vi "Usermgt.vi"(8 "error In":errorcluster) -> (0 "error out":errorcluster)   [LabVIEW 2015]
uses:
  Um- Save.ctl
  Um-Delete.ctl
  Um-Exit.ctl
  <vilib>/addons/database/Connection.llb/DB Tools Open Connec (String).vi
  <vilib>/addons/database/_DB Variant To Data/Database Variant To Data.xnode
  <vilib>/addons/database/NI_Database_API.lvlib
panel:
  out "data":variant[][](array[variant])
  in  "Operator Code":string
  out "error out 3":errorcluster
  out "User Name 2":string
  out "error out 2":errorcluster
  in  "Exit":T1
  in  "Deleat":T2
  in  "Save":T3
  in  "User Type":string
  in  "User Type":u16(ring) items=["Operator", "Supervisor", "admin"]
  in  "Re-Password":string
  in  "Password":string
  in  "User Name":string
  in  "User Table":i32(listbox)
  # "User Create"
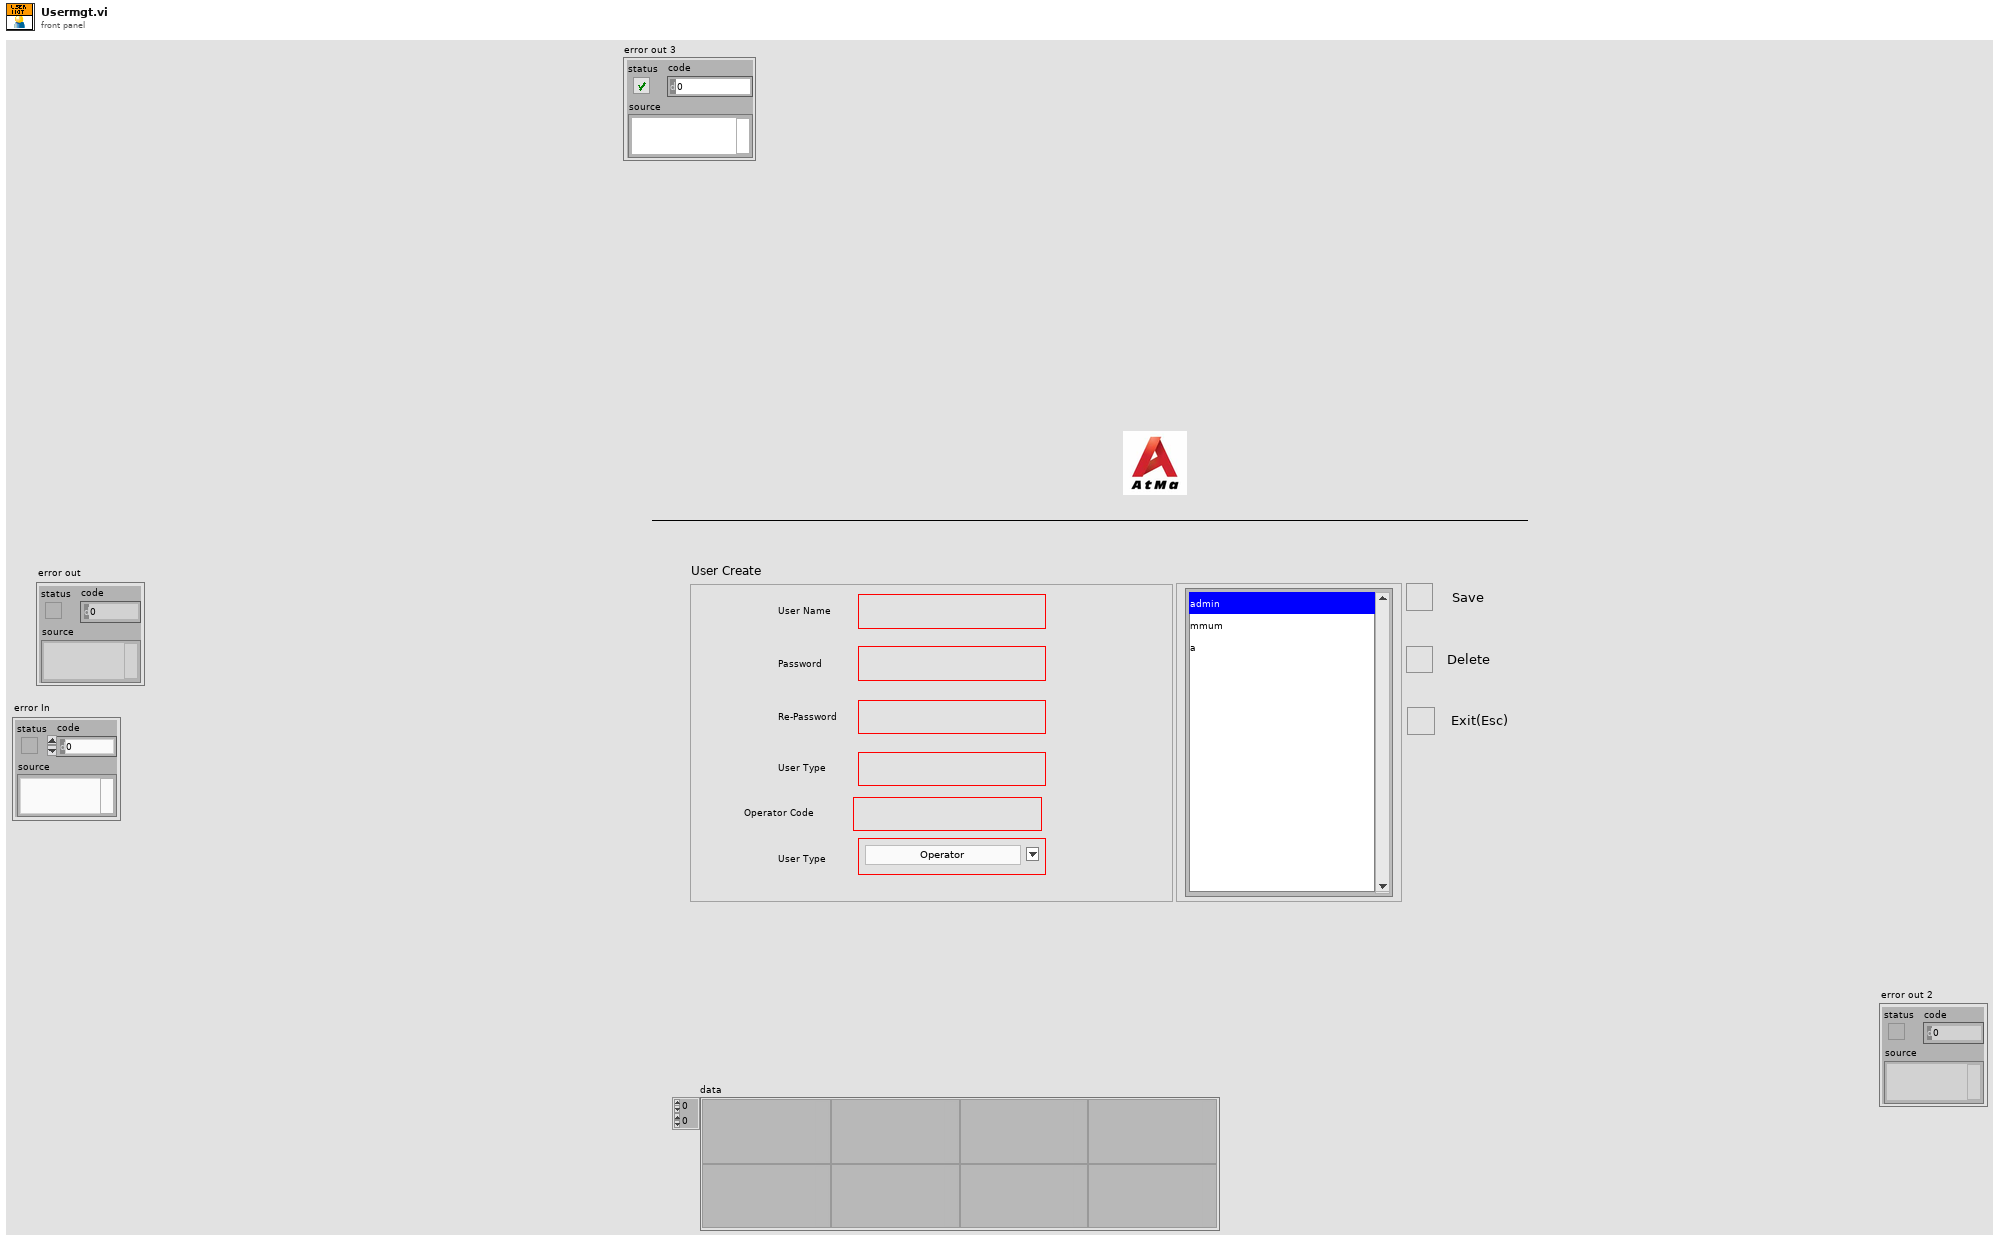
[diagram p1: front panel]
types:
  T1 = typedef "Um-Exit.ctl" = bool
  T2 = typedef "Um-Delete.ctl" = bool
  T3 = typedef "Um- Save.ctl" = bool
  T4 = cluster{"User Name":string, "Password":string, "User Type":string}
  T5 = typedef "NI_Database_API.lvlib/Conn ObjectReference.ctl" = refnum<k1>
  T6 = cluster{"User Name":string, "Password":string, "User Type":string, "Access right":string}
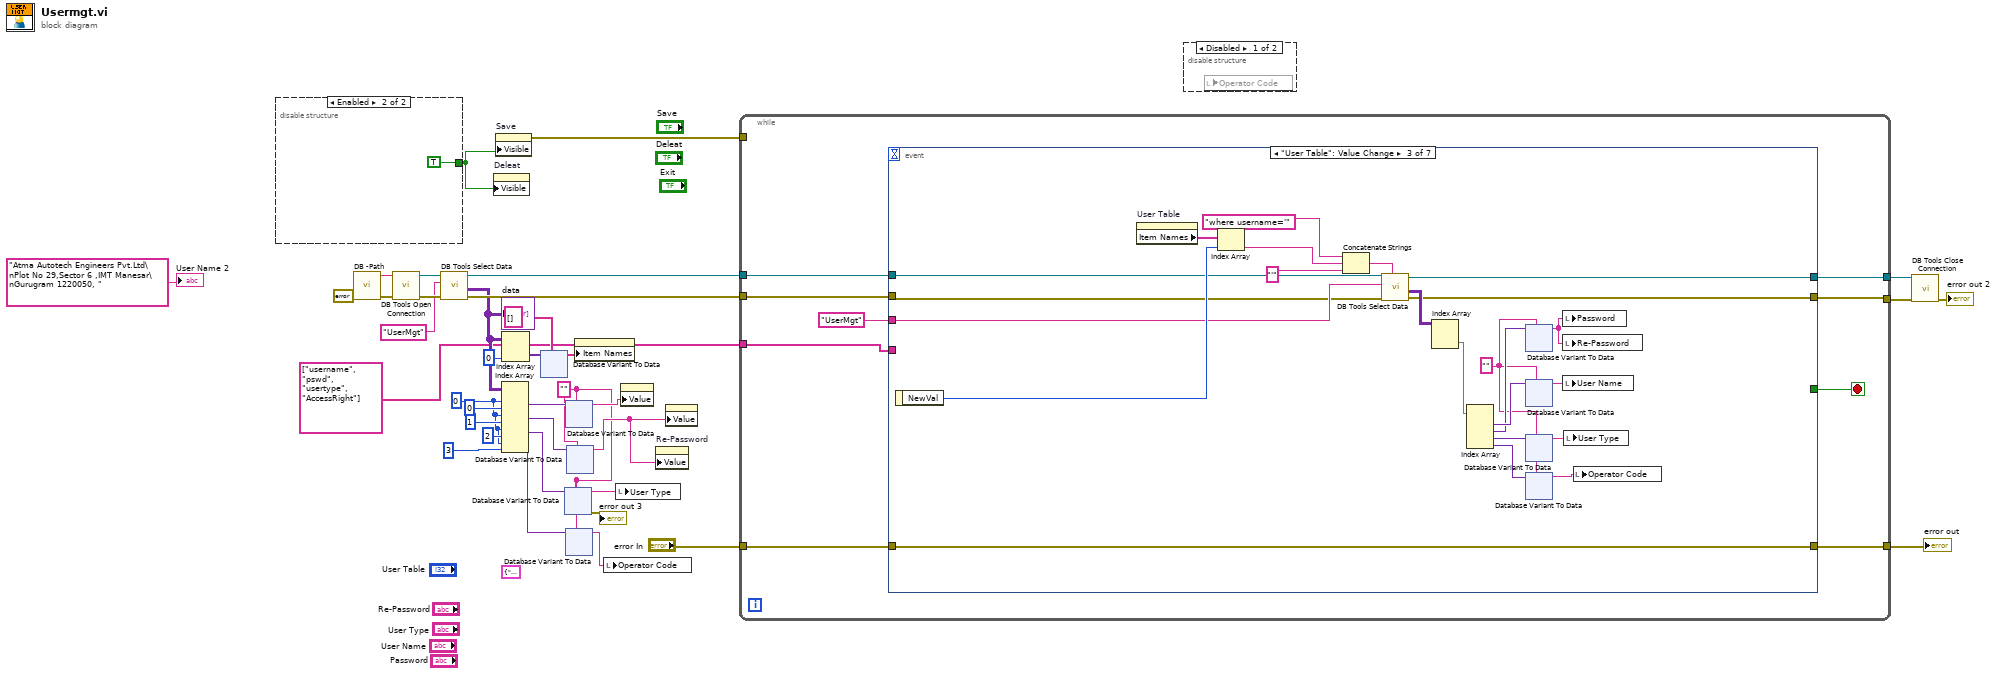
[diagram p0: block diagram]
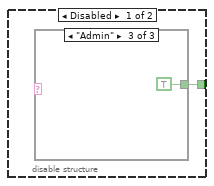
[diagram p3: hidden frame]
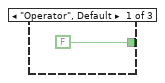
[diagram p4: hidden frame]
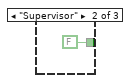
[diagram p5: hidden frame]
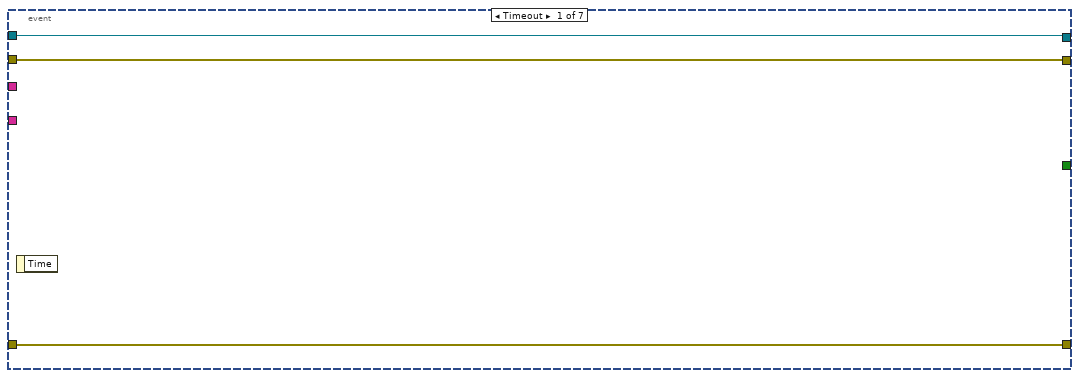
[diagram p6: hidden frame]
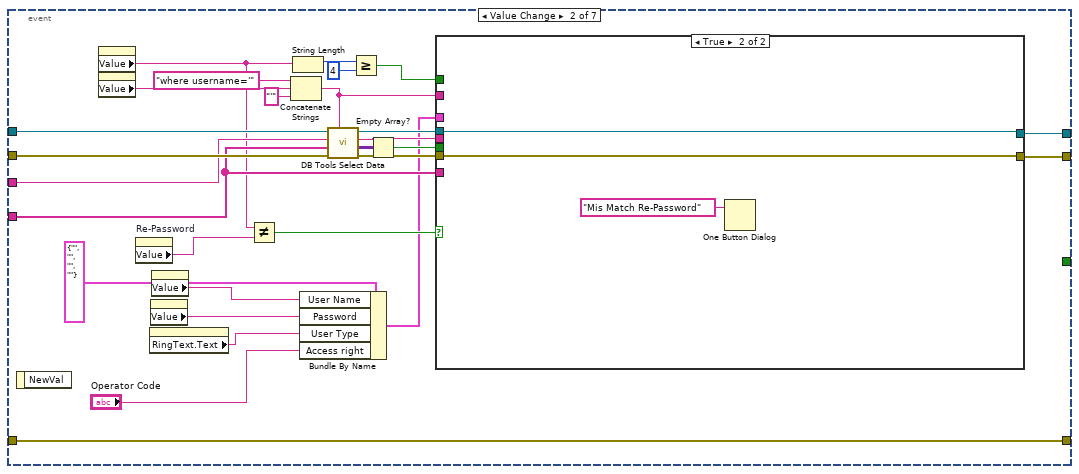
[diagram p7: hidden frame]
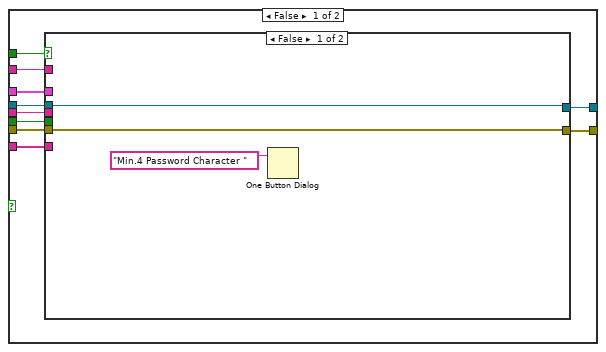
[diagram p8: hidden frame]
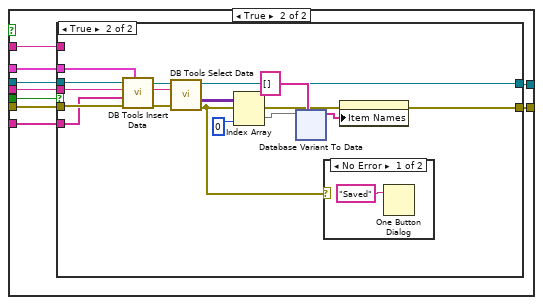
[diagram p9: hidden frame]
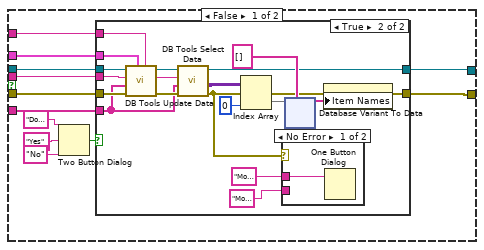
[diagram p10: hidden frame]
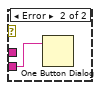
[diagram p12: hidden frame]
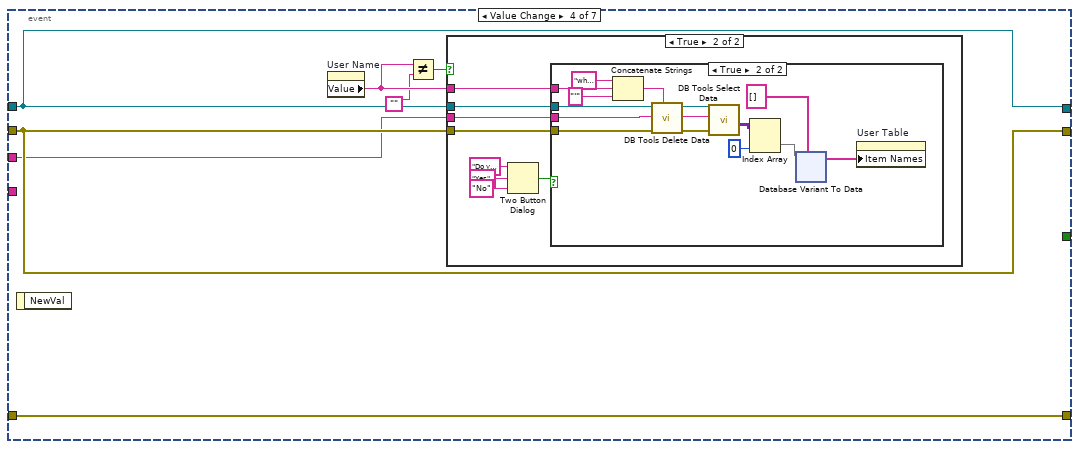
[diagram p14: hidden frame]
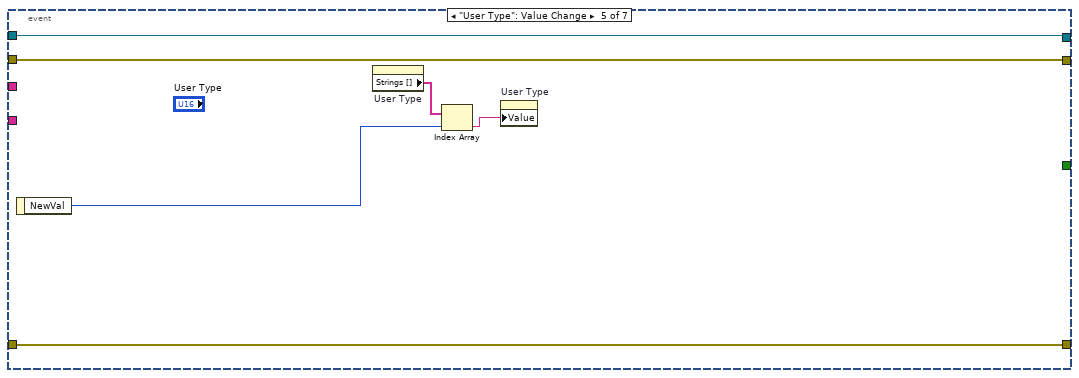
[diagram p17: hidden frame]
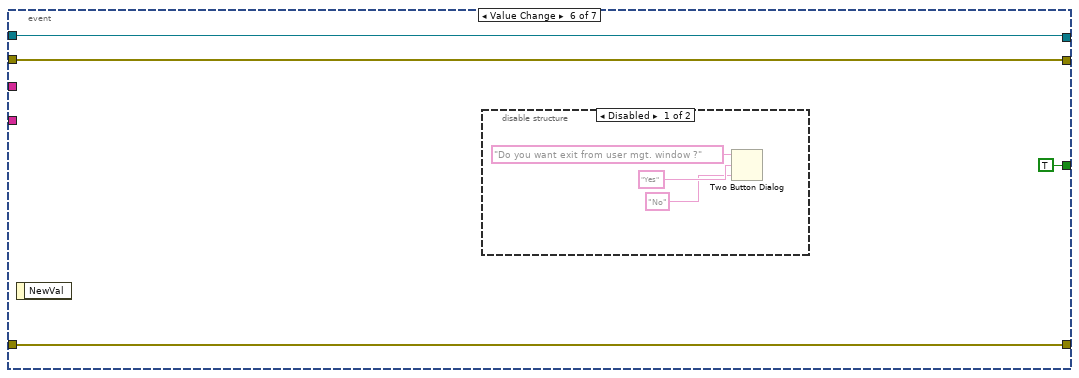
[diagram p18: hidden frame]
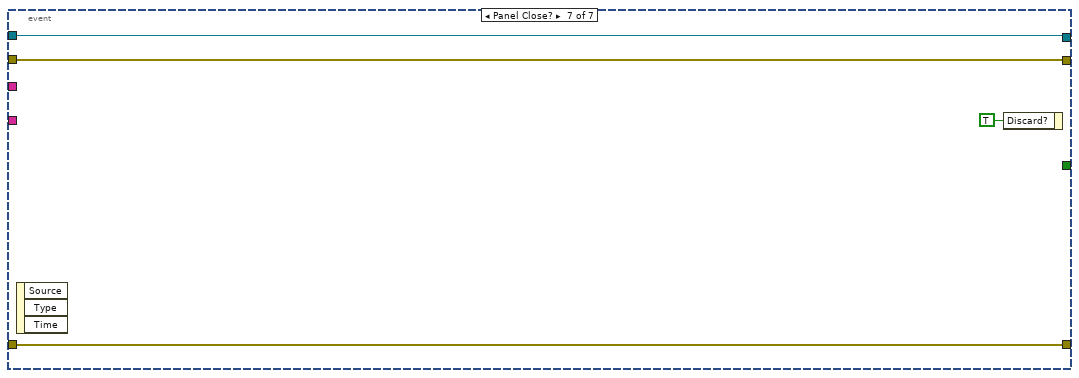
[diagram p20: hidden frame]
diagram:
  w2 = ""
  w4 = 0 ("index (row)")
  (unwired) T4 {"User Name"="", "Password"="", "User Type"=""} ("Input data")
  n1 = disable-structure shown="Enabled" {
    disable-tunnel: [w37 TRUE] -> w14
    frame Disabled {
      n2 = case shown="\"Admin\"" {
        selector: _ -> [_ _ _]
        tunnel: [FALSE FALSE TRUE] -> w37
        frame "Operator", Default {
        }
        frame "Supervisor" {
        }
        frame "Admin" {
        }
      }
    }
    frame Enabled {
    }
  }
  n3 = call "DB -Path.vi"() -> ("String"=w36:string)  [unwired: 11 in]
  n4 = call-poly <vilib>:"DB Tools Open Connection.vi"("error in (no error)"=errorcluster {"status"=FALSE, "code"=0, "source"=""}, "connection information"=w36) -> ("error out"=w33:errorcluster, "connection reference"=w32:T5)  [unwired: 6 in]
  n5 = call <vilib>:"DB Tools Select Data.vi"("error in (no error)"=w33, "table"="UserMgt", "connection reference"=w32) -> ("error out"=w30:errorcluster, "data"=w23:variant[][], "connection reference out"=w31:T5)  [unwired: 3 in]
  "data" <- w23
  n6 = property on="Deleat" class="Bool (strict)"("Visible"=w14) -> ()  [unwired: 2 in, 2 out]
  n7 = property on="Save" class="Bool (strict)"("Visible"=w14) -> (error out=w13:errorcluster)  [unwired: 2 in, 1 out]
  n8 = Index Array(array=w23, index (row) #1=w4, index (col) #1=0 ("disabled index (col)"), index (row) #2=w4, index (col) #2=1 ("disabled index (col)"), index (row) #3=w4, index (col) #3=2 ("disabled index (col)"), index (row) #4=w4, index (col) #4=3 ("index (col)")) -> (element #1=w24:variant, element #2=w20:variant, element #3=w16:variant, element #4=w3:variant)
  n9 = Index Array(array=w23, index (col)=0 ("disabled index (col)")) -> (element=w28:variant[])  [unwired: 1 in]
  n10 = xnode "Database Variant To Data"("database variant"=w28, "type"=string[] []) -> ("data"=w25:string[])  [unwired: 1 in, 1 out]
  n11 = xnode "Database Variant To Data"("database variant"=w16, "type"=w2) -> ("data"=w15:string, "error out"=→"error out 3":errorcluster)  [unwired: 1 in]
  n12 = xnode "Database Variant To Data"("database variant"=w24, "type"=w2) -> ("data"=w19:string)  [unwired: 1 in, 1 out]
  n13 = xnode "Database Variant To Data"("database variant"=w3, "type"=w2) -> ("data"=w1:string)  [unwired: 1 in, 1 out]
  n14 = xnode "Database Variant To Data"("database variant"=w20, "type"=w2) -> ("data"=w18:string)  [unwired: 1 in, 1 out]
  n15 = property on="User Table" class="LstBox (strict)"("Item Names"=w25) -> ()  [unwired: 2 in, 2 out]
  n16 = local write "Operator Code"(w1) -> ()
  n17 = local write "User Type"(w15) -> ()
  n18 = property on="User Name" class="Str"("Value"=w19) -> ()  [unwired: 2 in, 2 out]
  n19 = property on="Re-Password" class="Str"("Value"=w18) -> ()  [unwired: 2 in, 2 out]
  n20 = property on="Password" class="Str"("Value"=w18) -> ()  [unwired: 2 in, 2 out]
  n21 = while {
    tunnel: w31 -> [w49]
    tunnel: w30 -> [w48]
    tunnel: [w46] -> w35
    tunnel: [w45] -> w34
    tunnel: w13 -> [_]
    tunnel: string[] ["username", "pswd", "usertype", "AccessRight"] ("columns") -> [w44]
    tunnel: "error In" -> [w43]
    tunnel: [w42] -> w9
    stop <- w50 stop-if-true
    n22 = event shown="[2] \"User Table\": Value Change" {
      selector: _ -> [_ _ _ _ _ _ _]
      dyn-events: _ -> [_ _ _ _ _ _ _]
      timeout: _ -> [_ _ _ _ _ _ _]
      tunnel: [_ _ _ _ _ TRUE ("T button?") _] -> w50
      tunnel: w49 -> [w53 w80 w238 w387 w450 w457 w462]
      tunnel: w48 -> [w52 w79 w237 w386 w449 w456 w461]
      tunnel: "UserMgt" ("table") -> [_ w72 w246 w382 _ _ _]
      tunnel: w44 -> [_ w71 _ _ _ _ _]
      tunnel: [w53 w70 w236 w387 w450 w457 w462] -> w46
      tunnel: [w52 w69 w235 w386 w449 w456 w461] -> w45
      tunnel: w43 -> [w51 w55 w233 w381 w448 w454 w463]
      tunnel: [w51 w55 w233 w381 w448 w454 w463] -> w42
      event Timeout {
        n23 = event-data() -> ()  [unwired: 1 in, 1 out]
      }
      event Value Change {
        n24 = event-data() -> ()  [unwired: 1 in, 1 out]
        n25 = property on="Password" class="Str"() -> ("Value"=w57:string)  [unwired: 2 in, 2 out]
        n26 = property on="User Name" class="Str"() -> ("Value"=w56:string)  [unwired: 2 in, 2 out]
        n27 = property on="Re-Password" class="Str"() -> ("Value"=w63:string)  [unwired: 2 in, 2 out]
        n28 = property on="User Type" class="Ring (strict)"() -> ("RingText.Text"=w60:string)  [unwired: 2 in, 2 out]
        n29 = property on="Password" class="Str"() -> ("Value"=w62:string)  [unwired: 2 in, 2 out]
        n30 = property on="User Name" class="Str"() -> ("Value"=w61:string)  [unwired: 2 in, 2 out]
        n31 = Not Equal?(x=w57, y=w63) -> (x != y?=w64:bool)
        n32 = Concatenate Strings("where username='" ("condition"), w56, "'" ("User Name")) -> (w68:string)
        n33 = String Length(string=w57) -> (length=w67:i32)
        n34 = Bundle By Name(cluster=T6 {"User Name"="", "Password"="", "User Type"="", "Access right"=""} ("input cluster"), "User Name"=w61, "Password"=w62, "User Type"=w60, "Access right"="Operator Code") -> (w58:T6)
        n35 = call <vilib>:"DB Tools Select Data.vi"("condition"=w68, "error in (no error)"=w79, "columns"=w71, "table"=w72, "connection reference"=w80) -> ("error out"=w73:errorcluster, "data"=w78:variant[][], "connection reference out"=w74:T5)  [unwired: 1 in]
        n36 = Greater Or Equal?(x=w67, y=4) -> (x >= y?=w65:bool)
        n37 = Empty Array?(array=w78) -> (empty?=w77:bool)
        n38 = case shown="True" w64 {
          tunnel: w77 -> [w90 _]
          tunnel: w74 -> [w89 w229]
          tunnel: w73 -> [w88 w228]
          tunnel: w72 -> [w87 _]
          tunnel: w71 -> [w86 _]
          tunnel: w58 -> [w85 _]
          tunnel: [w84 w229] -> w70
          tunnel: [w83 w228] -> w69
          tunnel: w68 -> [w82 _]
          tunnel: w65 -> [w81 _]
          frame False {
            n39 = case shown="False" w81 {
              tunnel: w90 -> [_ w102]
              tunnel: w89 -> [w93 w101]
              tunnel: w88 -> [w92 w100]
              tunnel: w87 -> [_ w99]
              tunnel: w86 -> [_ w98]
              tunnel: w85 -> [_ w97]
              tunnel: [w93 w96] -> w84
              tunnel: [w92 w95] -> w83
              tunnel: w82 -> [_ w94]
              frame False {
                n40 = One Button Dialog(message="Min.4 Password Character ") -> ()  [unwired: 1 in, 1 out]
              }
              frame True {
                n41 = case shown="True" w102 {
                  tunnel: w101 -> [w114 w187]
                  tunnel: w100 -> [w113 w186]
                  tunnel: w99 -> [w108 w181]
                  tunnel: w98 -> [w105 w185]
                  tunnel: w97 -> [w106 w184]
                  tunnel: [w104 w175] -> w96
                  tunnel: [w103 w174] -> w95
                  tunnel: w94 -> [w107 _]
                  frame False {
                    n42 = Two Button Dialog(message="Do you want  modification" ("T button name (\"OK\")"), 1:"No" ("F button name (\"Cancel\")"), 2:"Yes" ("T button name (\"OK\")")) -> (T button?=w112:bool)
                    n43 = case shown="True" w112 {
                      tunnel: w114 -> [w116 w133]
                      tunnel: w113 -> [w115 w132]
                      tunnel: w108 -> [_ w127]
                      tunnel: w107 -> [_ w131]
                      tunnel: w106 -> [_ w130]
                      tunnel: w105 -> [_ w121]
                      tunnel: [w116 w120] -> w104
                      tunnel: [w115 w119] -> w103
                      frame False {
                      }
                      frame True {
                        n44 = call <vilib>:"DB Tools Update Data.vi"("condition"=w131, "data"=w130, "error in (no error)"=w132, "columns"=w121, "table"=w127, "connection reference"=w133) -> ("error out"=w128:errorcluster, "connection reference out"=w129:T5)  [unwired: 4 in]
                        n45 = call <vilib>:"DB Tools Select Data.vi"("error in (no error)"=w128, "columns"=w121, "table"=w127, "connection reference"=w129) -> ("error out"=w119:errorcluster, "data"=w126:variant[][], "connection reference out"=w120:T5)  [unwired: 2 in]
                        n46 = Index Array(array=w126, index (col)=0 ("disabled index (col)")) -> (element=w124:variant[])  [unwired: 1 in]
                        n47 = case shown="No Error" w119 {
                          tunnel: "Modification is Successfully" ("T button name (\"OK\")") -> [w134 _]
                          tunnel: "Modification is Unsuccessfully" ("T button name (\"OK\")") -> [_ w135]
                          frame No Error {
                            n48 = One Button Dialog(message=w134) -> ()  [unwired: 1 in, 1 out]
                          }
                          frame Error {
                            n49 = One Button Dialog(message=w135) -> ()  [unwired: 1 in, 1 out]
                          }
                        }
                        n50 = xnode "Database Variant To Data"("database variant"=w124, "type"=string[] []) -> ("data"=w122:string[])  [unwired: 1 in, 1 out]
                        n51 = property on="User Table" class="LstBox (strict)"("Item Names"=w122) -> ()  [unwired: 2 in, 2 out]
                      }
                    }
                  }
                  frame True {
                    n52 = call <vilib>:"DB Tools Insert Data.vi"("data"=w184, "error in (no error)"=w186, "columns"=w185, "table"=w181, "connection reference"=w187) -> ("error out"=w182:errorcluster, "connection reference out"=w183:T5)  [unwired: 5 in]
                    n53 = call <vilib>:"DB Tools Select Data.vi"("error in (no error)"=w182, "table"=w181, "connection reference"=w183) -> ("error out"=w174:errorcluster, "data"=w180:variant[][], "connection reference out"=w175:T5)  [unwired: 3 in]
                    n54 = Index Array(array=w180, index (col)=0 ("disabled index (col)")) -> (element=w178:variant[])  [unwired: 1 in]
                    n55 = xnode "Database Variant To Data"("database variant"=w178, "type"=string[] []) -> ("data"=w176:string[])  [unwired: 1 in, 1 out]
                    n56 = case shown="No Error" w174 {
                      frame No Error {
                        n57 = One Button Dialog(message="Saved" ("T button name (\"OK\")")) -> ()  [unwired: 1 in, 1 out]
                      }
                      frame Error {
                      }
                    }
                    n58 = property on="User Table" class="LstBox (strict)"("Item Names"=w176) -> ()  [unwired: 2 in, 2 out]
                  }
                }
              }
            }
          }
          frame True {
            n59 = One Button Dialog(message="Mis Match Re-Password") -> ()  [unwired: 1 in, 1 out]
          }
        }
      }
      event "User Table": Value Change {
        w230 = "" ("table")
        n60 = event-data() -> ("NewVal"=w250:i32)  [unwired: 1 in]
        n61 = property on="User Table" class="LstBox (strict)"() -> ("Item Names"=w251:string[])  [unwired: 2 in, 2 out]
        n62 = Index Array(array=w251, index=w250) -> (element=w248:string)
        n63 = Concatenate Strings("where username='" ("condition"), w248, "'" ("User Name")) -> (w247:string)
        n64 = call <vilib>:"DB Tools Select Data.vi"("condition"=w247, "error in (no error)"=w237, "table"=w246, "connection reference"=w238) -> ("error out"=w235:errorcluster, "data"=w245:variant[][], "connection reference out"=w236:T5)  [unwired: 2 in]
        n65 = Index Array(array=w245) -> (element=w244:variant[])  [unwired: 2 in]
        n66 = Index Array(array=w244) -> (element #1=w243:variant, element #2=w242:variant, element #3=w241:variant, element #4=w232:variant)  [unwired: 4 in]
        n67 = xnode "Database Variant To Data"("database variant"=w242, "type"=w230) -> ("data"=w239:string)  [unwired: 1 in, 1 out]
        n68 = xnode "Database Variant To Data"("database variant"=w243, "type"=w230) -> ("data"=w240:string)  [unwired: 1 in, 1 out]
        n69 = xnode "Database Variant To Data"("database variant"=w241, "type"=w230) -> ("data"=w234:string)  [unwired: 1 in, 1 out]
        n70 = xnode "Database Variant To Data"("database variant"=w232, "type"=w230) -> ("data"=w231:string)  [unwired: 1 in, 1 out]
        n71 = local write "Password"(w239) -> ()
        n72 = local write "Re-Password"(w239) -> ()
        n73 = local write "User Name"(w240) -> ()
        n74 = local write "User Type"(w234) -> ()
        n75 = local write "Operator Code"(w231) -> ()
      }
      event Value Change {
        n76 = event-data() -> ()  [unwired: 1 in, 1 out]
        n77 = property on="User Name" class="Str"() -> ("Value"=w385:string)  [unwired: 2 in, 2 out]
        n78 = Not Equal?(x=w385, y="") -> (x != y?=w383:bool)
        n79 = case shown="True" w383 {
          tunnel: w387 -> [_ w391]
          tunnel: w386 -> [_ w390]
          tunnel: w385 -> [_ w389]
          tunnel: w382 -> [_ w388]
          frame False {
          }
          frame True {
            n80 = Two Button Dialog(message="Do you want delete the user id & password", 1:"No" ("F button name (\"Cancel\")"), 2:"Yes" ("T button name (\"OK\")")) -> (T button?=w392:bool)
            n81 = case shown="True" w392 {
              tunnel: w391 -> [_ w409]
              tunnel: w390 -> [_ w408]
              tunnel: w389 -> [_ w404]
              tunnel: w388 -> [_ w401]
              frame False {
              }
              frame True {
                n82 = Concatenate Strings("where username='" ("condition"), w404, "'" ("User Name")) -> (w405:string)
                n83 = call <vilib>:"DB Tools Delete Data.vi"("condition"=w405, "error in (no error)"=w408, "table"=w401, "connection reference"=w409) -> ("error out"=w402:errorcluster, "connection reference out"=w403:T5)  [unwired: 6 in]
                n84 = call <vilib>:"DB Tools Select Data.vi"("error in (no error)"=w402, "table"=w401, "connection reference"=w403) -> ("data"=w399:variant[][])  [unwired: 3 in, 2 out]
                n85 = Index Array(array=w399, index (col)=0 ("disabled index (col)")) -> (element=w398:variant[])  [unwired: 1 in]
                n86 = xnode "Database Variant To Data"("database variant"=w398, "type"=string[] []) -> ("data"=w396:string[])  [unwired: 1 in, 1 out]
                n87 = property on="User Table" class="LstBox (strict)"("Item Names"=w396) -> ()  [unwired: 2 in, 2 out]
              }
            }
          }
        }
      }
      event "User Type": Value Change {
        n88 = event-data() -> ("NewVal"=w453:u16)  [unwired: 1 in]
        n89 = property on="User Type" class="Ring (strict)"() -> ("Strings []"=w452:string[])  [unwired: 2 in, 2 out]
        n90 = Index Array(array=w452, index=w453) -> (element=w451:string)
        n91 = property on="User Type" class="Str"("Value"=w451) -> ()  [unwired: 2 in, 2 out]
      }
      event Value Change {
        n92 = event-data() -> ()  [unwired: 1 in, 1 out]
        n93 = disable-structure shown="Disabled" {
          frame Disabled {
            n94 = Two Button Dialog(message="Do you want exit from user mgt. window ?", 1:"No" ("F button name (\"Cancel\")"), 2:"Yes" ("T button name (\"OK\")")) -> ()  [unwired: 1 out]
          }
          frame Enabled {
          }
        }
      }
      event Panel Close? {
        n95 = event-data() -> ()  [unwired: 1 in, 3 out]
        n96 = event-data("Discard?"=TRUE) -> ()  [unwired: 1 in, 1 out]
      }
    }
  }
  "error out" <- w9
  n97 = disable-structure shown="Disabled" {
    frame Disabled {
      n98 = local read "Operator Code"() -> ()  [unwired: 1 in]
    }
    frame Enabled {
    }
  }
  n99 = call <vilib>:"DB Tools Close Connection.vi"("error in (no error)"=w34, "connection reference"=w35) -> ("error out"=→"error out 2":errorcluster)  [unwired: 5 in]
  "User Name 2" <- "Atma Autotech Engineers Pvt.Ltd\nPlot No 29,Sector 6 ,IMT Manesar\nGurugram 1220050, " ("string")
